vi "PH_HamamatsuCamera.get cam settings.vi"(0 "i ref in":refnum<vi>, 1 "Cam Handle in":i32, 4 "Cam Error in":errorcluster, 5 "error in (no error)":errorcluster) -> (14 "i ref out":refnum<vi>, 15 "Handle out":i32, 18 "Cam Error out":errorcluster, 19 "error out":errorcluster)   [LabVIEW 2014, in "PH_HamamatsuCamera.lvlib"]
doc: "This VI gets several cam aquisition attributes, sets them to own attributes and the GUI elements."
uses:
  PH_HamamatsuCamera.lvlib
  PH_HamamatsuCamera.Cam Parameter.ctl
  PH_HamamatsuCamera.Parameter Set.ctl
panel:
  in  "Parameter":T1=4215968 items=["SENSOR MODE"=4212128, "CCD MODE"=4212384, "READOUT MODE"=4211872, "ACTIVE VIEW INDEX"=4343136, "BITS PER CHANNEL"=4342976, "IMAGE PIXEL TYPE"=4343296, "BINNING"=4215968, "EXPOSURE TIME"=2049184, "CONTRAST GAIN"=3163312, "CONTRAST OFFSET"=3163328, "LIGHT MODE"=2114720, "SENSITIVITY"=2114992, "PHOTON IMAGING MODE"=2115200, "HIGH DYNAMIC RANGE MODE"=3163360, "WHITE BALANCE"=3163568, "TEMPERATURE"=2115232, "TEMPERATURE TARGET"=2115264, "SENSOR COOLER FAN"=2115296, "LINEBUNDLE HEIGHT"=4212192, "MECHANICAL SHUTTER"=2115488, "BACK FOCUS POSITION"=8422304, "TRIGGER CONNECTOR"=1066432, "TRIGGER SOURCE"=1066144, "OUTPUT TRIGGER SOURCE"=1852576, "TRIGGER GLOBAL EXPOSURE"=2049680, "FIRST TRIGGER BEHAVIOR"=2049696, "CHANNEL SYNC"=1852352, "READOUT DIRECTION"=4211904, "PRE HSYNC COUNT"=1852704, "INTERNAL LINE SPEED"=4191408, "INTERNAL LINE INTERVAL"=4191424]
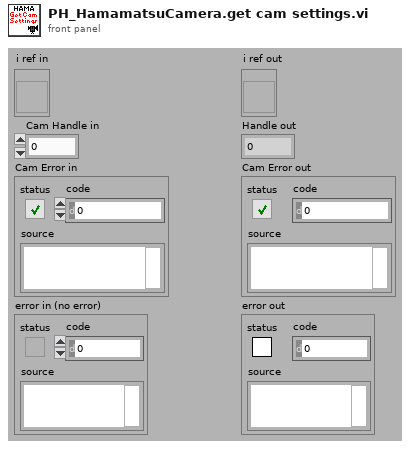
[diagram p1: front panel]
types:
  T1 = typedef "PH_HamamatsuCamera.lvlib/PH_HamamatsuCamera.Cam Parameter.ctl" = u32
  T2 = typedef "PH_HamamatsuCamera.lvlib/PH_HamamatsuCamera.i attribute.ctl" = cluster{"Gui Refs":cluster{"Camera Details":refnum<vi>, "ROI":refnum<vi>, "Set ROI to Maximum":refnum<vi>, "Trigger Parameters":refnum<vi>, "Brightness":refnum<vi>, "Shutter":refnum<vi>, "Gain":refnum<vi>, "Trigger Timeout":refnum<vi>, "Trigger Polarity":refnum<vi>, "Trigger Mode":refnum<vi>, "Parameters":refnum<vi>, "Set Cam Parameter":refnum<vi>, "Parameter to set":refnum<vi>, "Value to set":refnum<vi>}, "Cam":cluster{"Handle":i32, "Details":cluster{"Model":string, "Camera ID":string, "Firmware":string}, "Buffer Info":cluster{"height":u32, "width":u32, "datatype":u32}}, "H Offset":cluster{"Value":i32, "Minimum":i32, "Maximum":i32, "Increment":i32}, "V Offset":cluster{"Value":i32, "Minimum":i32, "Maximum":i32, "Increment":i32}, "H Width":cluster{"Value":i32, "Minimum":i32, "Maximum":i32, "Increment":i32}, "V Width":cluster{"Value":i32, "Minimum":i32, "Maximum":i32, "Increment":i32}, "Trigger Parameters":T3, "Trigger Timeout":u32, "Parameters":T4[], "Indicees Cam Parameters":cluster{"Brightness":i32, "Shutter":i32, "Gain":i32}, "Wanted Values":cluster{"Trigger Settings":T3[], "ROI":T5[], "Parameter":cluster{"Name":string, "Value":dbl}[]}}
  T3 = typedef "PH_HamamatsuCamera.lvlib/PH_HamamatsuCamera.Trigger Parameter.ctl" = cluster{"Mode":u32, "Polarity":u32, "Times":u32, "Delay":dbl}
  T4 = typedef "PH_HamamatsuCamera.lvlib/PH_HamamatsuCamera.Parameter Set.ctl" = cluster{"Parameter":string, "Value":dbl, "Writable":bool, "Range":cluster{"min":dbl, "max":dbl, "step":dbl}, "Default":dbl, "Value Names":cluster{"Name":string, "Value":dbl}[], "Text Values":bool}
  T5 = typedef "PH_HamamatsuCamera.lvlib/PH_HamamatsuCamera.ROI.ctl" = cluster{"Horizontal Offset":i32, "Vertical Offset":i32, "Horizontal Width":i32, "Vertical Width":i32}
  T6 = typedef "LVStringsAndValuesArrayTypeDef_U32.ctl" = cluster{"String":string, "Value":u32}[]
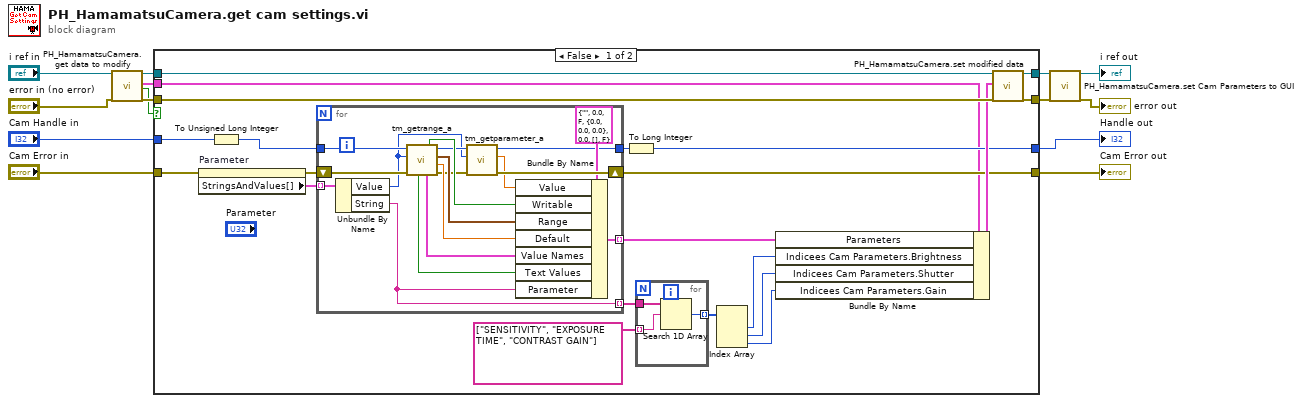
[diagram p0: block diagram]
diagram:
  n1 = call "PH_HamamatsuCamera.get data to modify.vi"("i ref in"="i ref in", "error in (no error)"="error in (no error)") -> ("i ref out"=w7:refnum<vi>, "i attribute"=w5:T2, "timed out"=w6:bool, "error out"=w8:errorcluster)  [unwired: 14 in]
  n2 = case shown="False" w6 {
    tunnel: w8 -> [w35 w58]
    tunnel: [w22 w58] -> w1
    tunnel: w7 -> [w34 w59]
    tunnel: [w23 w59] -> w3
    tunnel: w5 -> [w19 _]
    tunnel: "Cam Handle in" -> [w26 w57]
    tunnel: "Cam Error in" -> [w31 w56]
    tunnel: [w28 w56] -> w10
    tunnel: [w24 w57] -> w9
    frame False {
      n3 = property on="Parameter" class="Ring (strict)"(error in=w31) -> (error out=w30:errorcluster, "StringsAndValues[]"=w29:T6)  [unwired: 1 in, 1 out]
      n4 = To Unsigned Long Integer(number=w26) -> (unsigned 32bit integer=w25:u32)
      n5 = for {
        tunnel: [w55] -> w33 mode=indexing
        tunnel: w25 -> [w53]
        shift-right: [w46] -> w28
        shift-left: w30 -> [w54]
        tunnel: w29 -> [w43] mode=indexing
        tunnel: [w40] -> w27
        tunnel: [w39] -> w20 mode=indexing
        n6 = Unbundle By Name(w43) -> ("Value"=w42:u32, "String"=w39:string)
        n7 = call <userlib>:"tm_getrange_a.vi"("error in (no error)"=w54, "Parameter"=w42, "Handle in"=w53) -> ("error out"=w47:errorcluster, "default"=w50:dbl, "Range"=w51:cluster{"min":dbl, "max":dbl, "step":dbl}, "Handle out"=w45:u32, "Value Names"=w49:cluster{"Name":string, "Value":dbl}[], "Writable"=w52:bool, "Text Values"=w48:bool)  [unwired: 2 in]
        n8 = call <userlib>:"tm_getparameter_a.vi"("error in (no error)"=w47, "Parameter"=w42, "Handle in"=w45) -> ("error out"=w46:errorcluster, "Value out"=w44:dbl, "Handle out"=w40:u32)  [unwired: 6 in]
        n9 = Bundle By Name(cluster=T4 {"Parameter"="", "Value"=0.0, "Writable"=FALSE, "Range"={"min"=0.0, "max"=0.0, "step"=0.0}, "Default"=0.0, "Value Names"=[], "Text Values"=FALSE} ("Parameter Set"), "Value"=w44, "Writable"=w52, "Range"=w51, "Default"=w50, "Value Names"=w49, "Text Values"=w48, "Parameter"=w39) -> (w55:T4)
      }
      n10 = To Long Integer(number=w27) -> (32bit integer=w24:i32)
      n11 = for {
        tunnel: string[] ["SENSITIVITY", "EXPOSURE TIME", "CONTRAST GAIN"] -> [w37] mode=indexing
        tunnel: w20 -> [w38]
        tunnel: [w36] -> w21 mode=indexing
        n12 = Search 1D Array(1D array=w38, element=w37) -> (index of element=w36:i32)  [unwired: 1 in]
      }
      n13 = Index Array(array=w21) -> (element #1=w18:i32, element #2=w17:i32, element #3=w16:i32)  [unwired: 3 in]
      n14 = Bundle By Name(cluster=w19, "Parameters"=w33, "Indicees Cam Parameters.Brightness"=w18, "Indicees Cam Parameters.Shutter"=w17, "Indicees Cam Parameters.Gain"=w16) -> (w32:T2)
      n15 = call "PH_HamamatsuCamera.set modified data.vi"("i ref in"=w34, "i attribute"=w32, "error in (no error)"=w35) -> ("i ref out"=w23:refnum<vi>, "error out"=w22:errorcluster)  [unwired: 15 in]
    }
    frame True {
    }
  }
  "Cam Error out" <- w10
  "Handle out" <- w9
  n16 = call "PH_HamamatsuCamera.set Cam Parameters to GUI.vi"("i ref in"=w3, "error in (no error)"=w1) -> ("VI out"=→"i ref out":refnum<vi>, "error out"=→"error out":errorcluster)  [unwired: 16 in]
